vi "Make FileName.vi"(11 "Meas Name":string) -> (3 "Path":path)   [LabVIEW 2017]
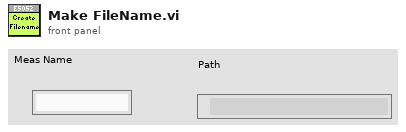
[diagram p1: front panel]
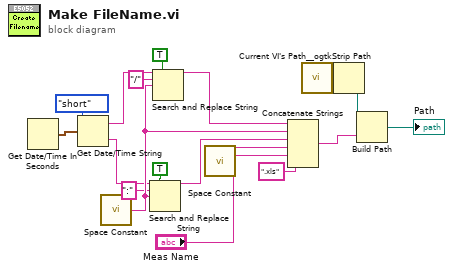
[diagram p0: block diagram]
diagram:
  n1 = Get Date/Time In Seconds() -> (seconds since 1Jan1904=w5:timestamp)
  n2 = Get Date/Time String(date format (0)=enum16{"short", "long", "abbreviated"}."short", seconds (now)=w5) -> (date string=w6:string, time string=w8:string)  [unwired: 1 in]
  n3 = call <vilib>:"Space Constant.vi"() -> ("String"=w14:string)
  n4 = Search and Replace String(replace all?=TRUE ("replace all? (F)"), input string=w8, search string=":", replace string=w14) -> (result string=w13:string)  [unwired: 4 in, 3 out]
  n5 = Search and Replace String(replace all?=TRUE ("replace all? (F)"), input string=w6, search string="/", replace string=w14) -> (result string=w12:string)  [unwired: 4 in, 3 out]
  n6 = call <vilib>:"Space Constant.vi"() -> ("String"=w1:string)
  n7 = Concatenate Strings(w12, w14, w13, w1, "Meas Name", ".xls" ("string")) -> (w15:string)
  n8 = call <userlib>:"Current VI's Path__ogtk.vi"() -> ("Current VI's Path (+ Relative)"=w18:path)  [unwired: 1 in]
  n9 = Strip Path(path=w18) -> (stripped path=w17:path)  [unwired: 1 out]
  n10 = Build Path(base path=w17, name or relative path=w15) -> (appended path=→"Path":path)
